vi "Read Alpha Value.vi"(8 "error in (no error)":errorcluster, 11 "SA in":refnum<class "SA.lvclass">) -> (0 "error out":errorcluster, 2 "Alpha Value":dbl, 3 "SA out":refnum<class "SA.lvclass">)   [LabVIEW 2013, in "SA.lvclass"]
uses:
  SA.lvclass
  SA.lvclass/SA.ctl
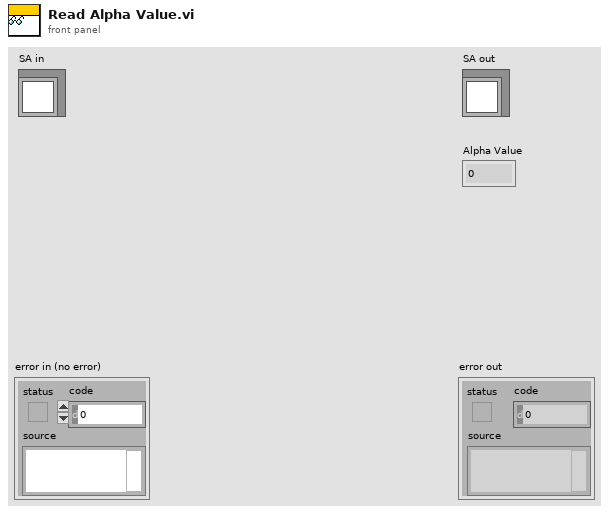
[diagram p1: front panel]
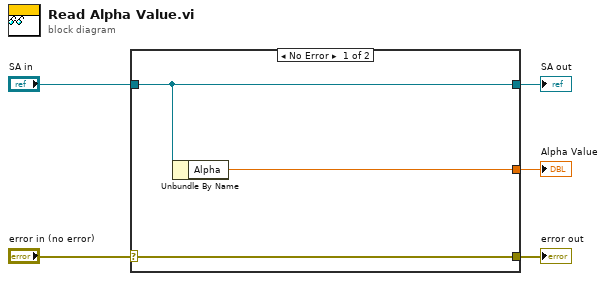
[diagram p0: block diagram]
diagram:
  n1 = case shown="No Error" "error in (no error)" {
    selector: "error in (no error)" -> [w8 w9]
    tunnel: [w8 w9] -> w4
    tunnel: [w7 w10] -> w2
    tunnel: "SA in" -> [w7 w10]
    tunnel: [w6 _] -> w1
    frame No Error {
      n2 = Unbundle By Name(w7) -> ("Alpha"=w6:dbl)
    }
    frame Error {
    }
  }
  "error out" <- w4
  "SA out" <- w2
  "Alpha Value" <- w1
